vi "roller_calc.vi"(11 "Roller Inputs":T4) -> (3 "Roller_Outputs":T2)   [LabVIEW 2013]
uses:
  roller_inputs.ctl
  roller_outputs.ctl
  <vilib>/Rock Robotics/WPI/Solenoid/WPI_SolenoidValue.ctl
  flinger/flinger_inputs.ctl
panel:
  in  "Flinger Inputs":T1
  in  "Roller_Outputs 2":T2
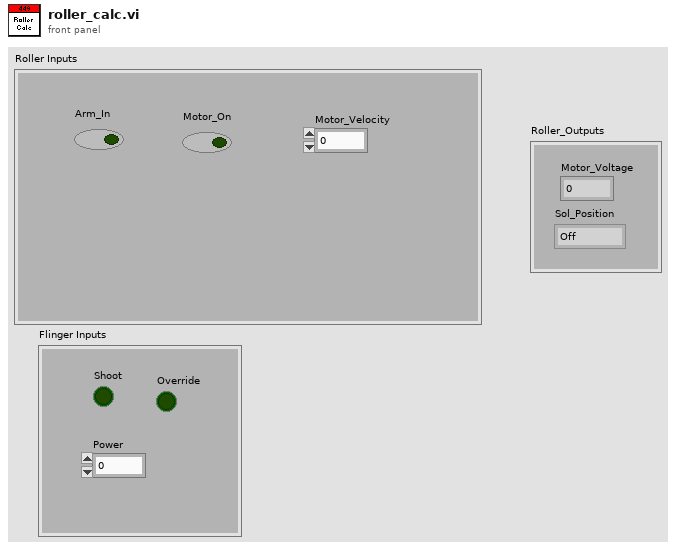
[diagram p1: front panel]
types:
  T1 = typedef "flinger_inputs.ctl" = cluster{"Shoot":bool, "Power":dbl, "Override":bool}
  T2 = typedef "roller_outputs.ctl" = cluster{"Sol_Position":T3, "Motor_Voltage":dbl}
  T3 = typedef "WPI_SolenoidValue.ctl" = enum16{"Off", "On", "Forward", "Reverse"}
  T4 = typedef "roller_inputs.ctl" = cluster{"Arm_In":bool, "Motor_On":bool, "Motor_Velocity":dbl}
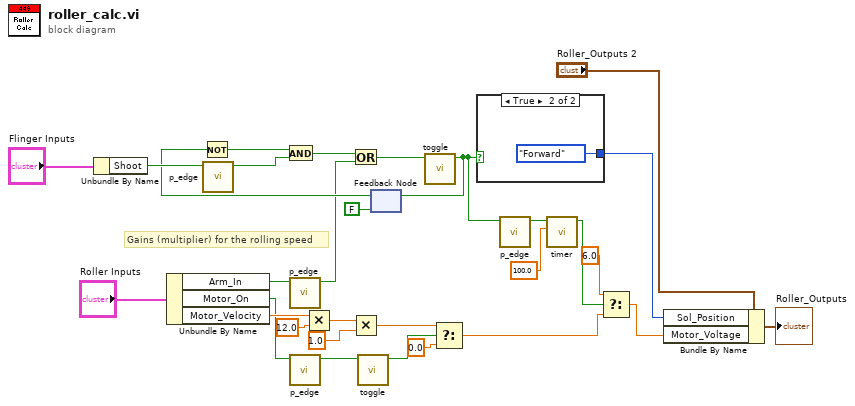
[diagram p0: block diagram]
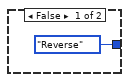
[diagram p2: hidden frame]
diagram:
  # "Gains (multiplier) for the rolling speed"
  n1 = Unbundle By Name("Flinger Inputs") -> ("Shoot"=w22:bool)
  n2 = Unbundle By Name("Roller Inputs") -> ("Arm_In"=w21:bool, "Motor_On"=w12:bool, "Motor_Velocity"=w20:dbl)
  n3 = call "p_edge.vi"("In"=w22) -> ("Out"=w16:bool)  [unwired: 10 in]
  n4 = call "p_edge.vi"("In"=w21) -> ("Out"=w14:bool)  [unwired: 10 in]
  n5 = call "p_edge.vi"("In"=w12) -> ("Out"=w11:bool)  [unwired: 10 in]
  n6 = Multiply(x=w20, y=12.0) -> (x*y=w25:dbl)
  n7 = Multiply(x=w25, y=1.0) -> (x*y=w9:dbl)
  n8 = call "toggle.vi"("In"=w11) -> ("Out"=w10:bool)  [unwired: 10 in]
  n9 = feedback #1(FALSE ("Out")) -> (w17:bool)
  n10 = Not(x=w17) -> (.not. x?=w18:bool)
  n11 = And(x=w18, y=w16) -> (x .and. y?=w13:bool)
  n12 = Or(x=w13, y=w14) -> (x .or. y?=w15:bool)
  n13 = call "toggle.vi"("In"=w15) -> ("Out"=w1:bool)  [unwired: 10 in]
  n14 = feedback-in #1(w1) -> ()
  n15 = Select(t=w9, s=w10, f=0.0) -> (s? t:f=w4:dbl)
  n16 = case shown="True" w1 {
    tunnel: [WPI_SolenoidValue."Reverse" ("Value") WPI_SolenoidValue."Forward" ("Value")] -> w27
    frame False {
    }
    frame True {
    }
  }
  n17 = call "p_edge.vi"("In"=w1) -> ("Out"=w7:bool)  [unwired: 10 in]
  n18 = call "timer.vi"("Time"=100.0, "Set"=w7) -> ("Out"=w5:bool)  [unwired: 9 in]
  n19 = Select(t=6.0, s=w5, f=w4) -> (s? t:f=w3:dbl)
  n20 = Bundle By Name(cluster="Roller_Outputs 2", "Sol_Position"=w27, "Motor_Voltage"=w3) -> (→"Roller_Outputs":T2)
